vi "Execute.vi"(6 "Index [-1]":i32=-1, 7 "Composite Object":refnum<class "CConfig Object.lvclass">, 8 "error in (no error)":errorcluster, 9 "Results":string[][](array[string]), 11 "Config Query in":refnum<class "Add Results Query.lvclass">) -> (0 "error out":errorcluster, 1 "Results":string[][](array[string]), 2 "Result":bool, 3 "Config Query out":refnum<class "Add Results Query.lvclass">, 4 "Index":i32, 5 "Composite Object":refnum<class "CConfig Object.lvclass">)   [LabVIEW 2013, in "Add Results Query.lvclass"]
doc: "Copyright 2018, Carya Automatisering, Wiebe Walstra."
uses:
  Add Results Query.lvclass
  CConfig Object.lvclass
  Add Results Query.lvclass/Add Results Query.ctl
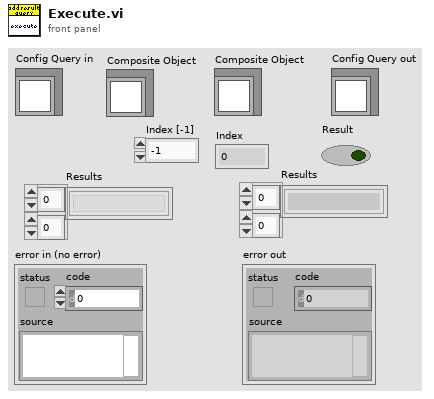
[diagram p1: front panel]
types:
  T1 = typedef "CConfig Object.lvclass/Data.ctl" = enum16{"pre", "name", "middle", "value", "post", "newline", "persistant", "tagged", "type"}
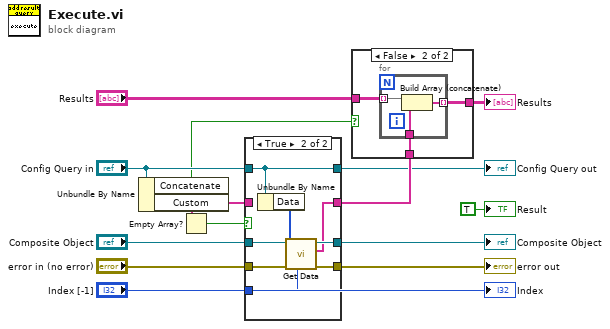
[diagram p0: block diagram]
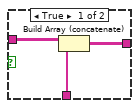
[diagram p3: hidden frame]
diagram:
  n1 = Unbundle By Name("Config Query in") -> ("Concatenate"=w3:bool, "Custom"=w2:string[])
  n2 = Empty Array?(array=w2) -> (empty?=w1:bool)
  n3 = case shown="True" w1 {
    tunnel: "error in (no error)" -> [w15 w26]
    tunnel: [w15 w25] -> w12
    tunnel: "Index [-1]" -> [_ w24]
    tunnel: "Composite Object" -> [w16 w23]
    tunnel: [w16 w22] -> w9
    tunnel: [w17 w21] -> w8
    tunnel: "Config Query in" -> [w18 w19]
    tunnel: [w18 w19] -> w4
    tunnel: w2 -> [w17 _]
    frame False {
    }
    frame True {
      n4 = Unbundle By Name(w19) -> ("Data"=w20:T1[])
      n5 = call-dynamic "Get Data.vi"("Index in"=w24, "error in (no error)"=w26, "Data"=w20, "Composite Object in"=w23) -> ("error out"=w25:errorcluster, "Data"=w21:string[], "Composite Object out"=w22:refnum<class "CConfig Object.lvclass">)  [unwired: 5 in]
    }
  }
  "error out" <- w12
  "Config Query out" <- w4
  "Composite Object" <- w9
  n6 = case shown="False" w3 {
    tunnel: "Results" -> [w29 w32]
    tunnel: w8 -> [w27 w30]
    tunnel: [w28 w31] -> w6
    frame True {
      n7 = Build Array (concatenate)(w29, w27) -> (w28:string[][])
    }
    frame False {
      n8 = for {
        tunnel: w32 -> [w35] mode=indexing
        tunnel: [w34] -> w31 mode=indexing
        tunnel: w30 -> [w33]
        n9 = Build Array (concatenate)(w35, w33) -> (w34:string[])
      }
    }
  }
  "Results" <- w6
  "Result" <- TRUE ("Result")
  "Index" <- "Index [-1]"
